vi "io.visa.init.vi"(8 "error in (no error)":errorcluster, 10 "Init Params":T1={"baud rate"=115200, "parity"=enum."None", "flow control"=0, "data bits"=8, "stop bits"=10, "msTimeout"=50, "Termination Char"="}", "End Read Mode"=2} {"baud rate" items=["75"=75, "110"=110, "134"=134, "150"=150, "300"=300, "600"=600, "1200"=1200, "1800"=1800, "2400"=2400, "4800"=4800, "7200"=7200, "9600"=9600, "14400"=14400, "19200"=19200, "28800"=28800, "38400"=38400, "56000"=56000, "57600"=57600, "115200"=115200, "128000"=128000, "230400"=230400]; "flow control" items=["None"=0, "XON/XOFF"=1, "RTS/CTS"=2, "DTR/DSR"=4]; "stop bits" items=["1.0"=10, "1.5"=15, "2.0"=20]; "End Read Mode" items=["None", "Last Bit", "TermChar"]}, 11 "VISA Refnum in":refnum<visa-resource-name>) -> (0 "error out":errorcluster, 3 "VISA Refnum out":refnum<visa-resource-name>)   [LabVIEW 2024]
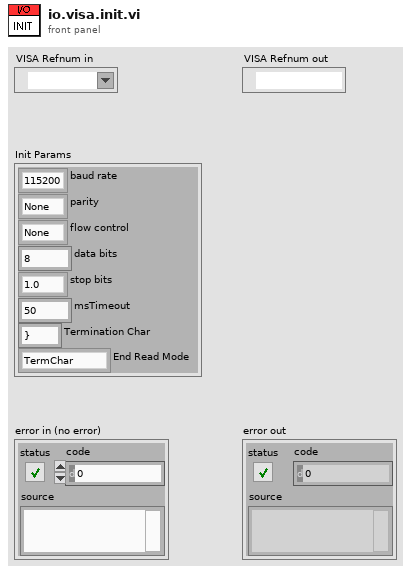
[diagram p1: front panel]
types:
  T1 = cluster{"baud rate":u32, "parity":enum16{"None", "Odd", "Even", "Mark", "Space"}, "flow control":u16, "data bits":u16, "stop bits":u16, "msTimeout":u32, "Termination Char":string, "End Read Mode":u16}
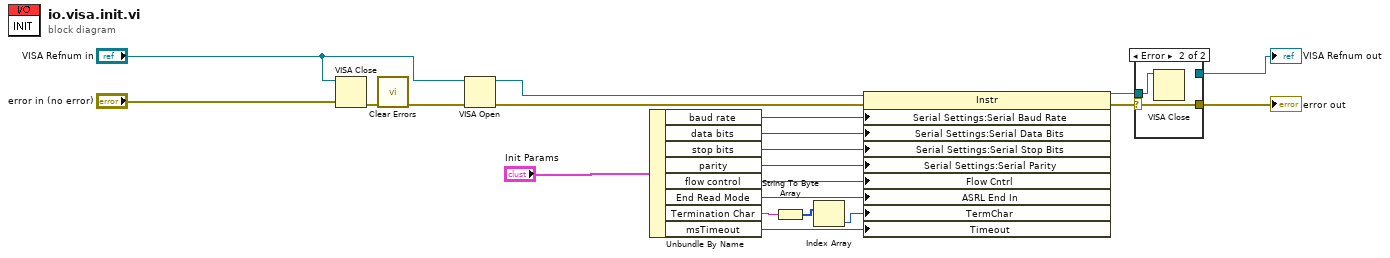
[diagram p0: block diagram]
diagram:
  n1 = VISA Close(VISA resource name="VISA Refnum in", error in (no error)="error in (no error)") -> (error out=w13:errorcluster)
  n2 = call <vilib>:"Clear Errors.vi"("error in (no error)"=w13) -> ("error out"=w12:errorcluster)  [unwired: 5 in, 1 out]
  n3 = VISA Open(error in (no error)=w12, VISA resource name="VISA Refnum in") -> (VISA resource name=w15:refnum<visa-resource-name>, error out=w16:errorcluster)  [unwired: 3 in]
  n4 = Unbundle By Name("Init Params") -> ("baud rate"=w5:u32, "data bits"=w11:u16, "stop bits"=w10:u16, "parity"=w9:enum16{"None", "Odd", "Even", "Mark", "Space"}, "flow control"=w6:u16, "End Read Mode"=w2:u16, "Termination Char"=w7:string, "msTimeout"=w1:u32)
  n5 = String To Byte Array(string=w7) -> (unsigned byte array=w8:u8[])
  n6 = Index Array(array=w8) -> (element=w3:u8)  [unwired: 1 in]
  n7 = property class="Instr"(reference=w15, error in=w16, "Serial Settings:Serial Baud Rate"=w5, "Serial Settings:Serial Data Bits"=w11, "Serial Settings:Serial Stop Bits"=w10, "Serial Settings:Serial Parity"=w9, "Flow Cntrl"=w6, "ASRL End In"=w2, "TermChar"=w3, "Timeout"=w1) -> (reference out=w14:refnum<visa-resource-name>, error out=w4:errorcluster)
  n8 = case shown="Error" w4 {
    selector: w4 -> [w22 w24]
    tunnel: w14 -> [w23 w25]
    tunnel: [w23 _] -> w18
    tunnel: [w22 w24] -> w19
    frame No Error {
    }
    frame Error {
      n9 = VISA Close(VISA resource name=w25) -> ()  [unwired: 1 in, 1 out]
    }
  }
  "error out" <- w19
  "VISA Refnum out" <- w18
